vi "SC-BG-formarraySD.vi"(1 "II channel seq":T1, 2 "I channel seq":T1) -> (0 "output array":dbl[][](array[numeric]))   [LabVIEW 2015]
uses:
  controls/data-cluster.ctl
  globalVarSD.vi
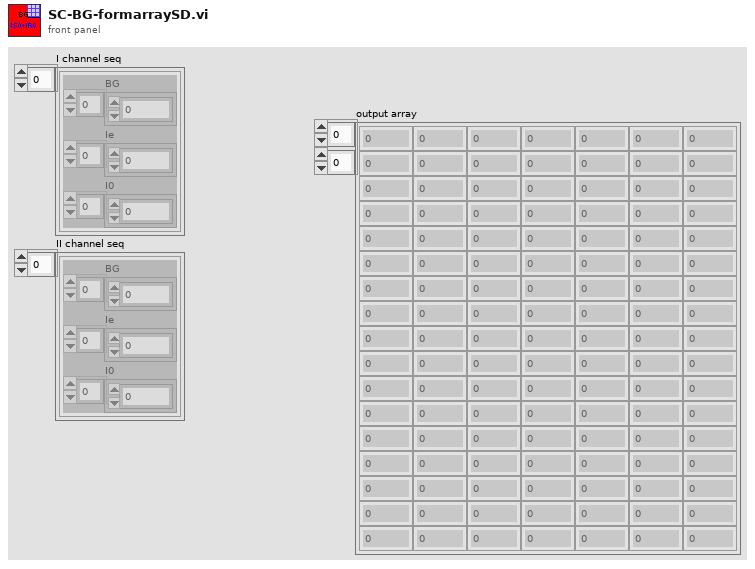
[diagram p1: front panel]
types:
  T1 = typedef "data-cluster.ctl" = cluster{"BG":i32[], "Ie":i32[], "I0":i32[]}[]
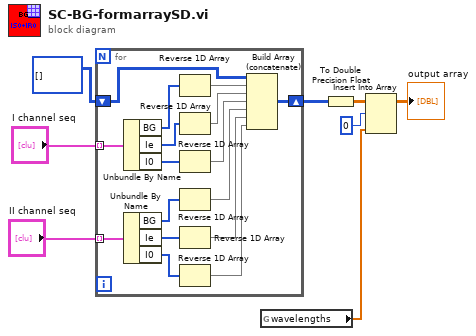
[diagram p0: block diagram]
diagram:
  n1 = for {
    tunnel: "I channel seq" -> [w24] mode=indexing
    tunnel: "II channel seq" -> [w23] mode=indexing
    shift-right: [w16] -> w2
    shift-left: i32[][] [] -> [w15]
    n2 = Unbundle By Name(w24) -> ("BG"=w21:i32[], "Ie"=w20:i32[], "I0"=w14:i32[])
    n3 = Unbundle By Name(w23) -> ("BG"=w22:i32[], "Ie"=w19:i32[], "I0"=w12:i32[])
    n4 = Reverse 1D Array(array=w21) -> (reversed array=w18:i32[])
    n5 = Reverse 1D Array(array=w20) -> (reversed array=w17:i32[])
    n6 = Reverse 1D Array(array=w14) -> (reversed array=w13:i32[])
    n7 = Reverse 1D Array(array=w22) -> (reversed array=w11:i32[])
    n8 = Reverse 1D Array(array=w19) -> (reversed array=w10:i32[])
    n9 = Reverse 1D Array(array=w12) -> (reversed array=w9:i32[])
    n10 = Build Array (concatenate)(w15, w18, w17, w13, w11, w10, w9) -> (w16:i32[][])
  }
  n11 = global read "globalVarSD.vi" "wavelengths"() -> (w4:dbl[])
  n12 = To Double Precision Float(number=w2) -> (double precision float=w1:dbl[][])
  n13 = Insert Into Array(array=w1, index (row)=0, new element=w4) -> (→"output array":dbl[][])  [unwired: 1 in]
